vi "Web URLs.vi"() -> (2 "Index":string, 3 "Base":string="https://lvgpack.com")   [LabVIEW 2020, in "GPack.lvlib"]
uses:
  GPack.lvlib
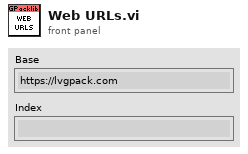
[diagram p1: front panel]
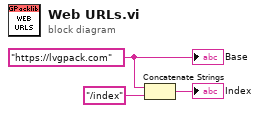
[diagram p0: block diagram]
diagram:
  w3 = "https://lvgpack.com"
  n1 = Concatenate Strings(w3, "/index" ("string")) -> (→"Index":string)
  "Base" <- w3
